vi "Pub.global.vi"() -> ()   [LabVIEW 2014]
uses:
  <vilib>/addons/zeromq/zmq_socket.lvclass
  <vilib>/addons/zeromq/zmq_context.lvclass
panel:
  in  "Pub":T1
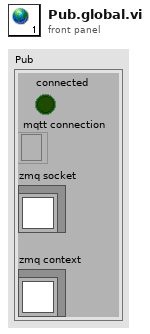
[diagram p1: front panel]
types:
  T1 = cluster{"zmq socket":refnum<class "zmq_socket.lvclass">, "mqtt connection":refnum<k5>, "zmq context":refnum<class "zmq_context.lvclass">, "connected":bool}
diagram:
